vi "Save Issue Global.vi"(11 "output cluster":cluster{"path":path, "error out":errorcluster}) -> ()   [LabVIEW 2013]
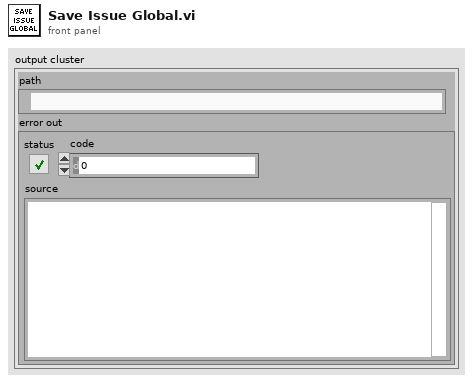
[diagram p1: front panel]
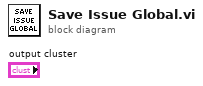
[diagram p0: block diagram]
diagram:
